vi "draw_time_stamp.vi"(8 "error in (no error)":errorcluster, 11 "Image in":refnum<class "Image.lvclass">) -> (0 "error out":errorcluster, 3 "Image out":refnum<class "Image.lvclass">)   [LabVIEW 2010, in "Image.lvclass"]
uses:
  Image.lvclass
  <vilib>/vision/Image Controls.llb/IMAQ Image.ctl
  ErrorController/ErrorController/class_data.vi
  ErrorController/ErrorController/ErrorController.lvclass
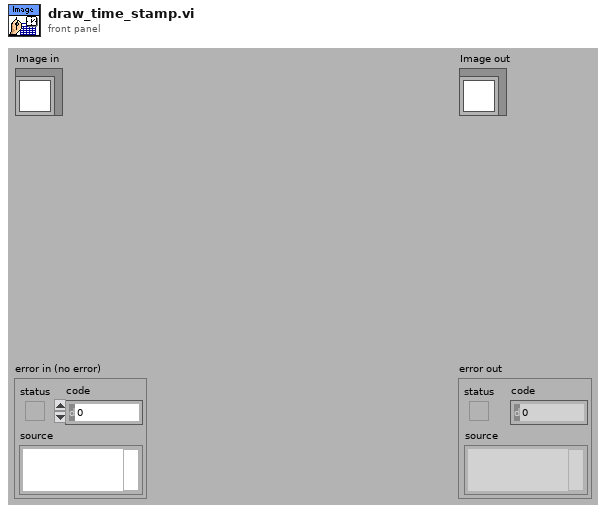
[diagram p1: front panel]
types:
  T1 = cluster{"Desired Font (Application)":enum16{"User-specified Font", "Application Font", "System Font", "Dialog Font"}, "[User-specified Font]":cluster{"Font Name":string, "Size":i16, "Strikeout?":bool, "Italic?":bool, "Underline?":bool, "Outline?":bool, "Shadow?":bool, "Bold?":bool, "Rotation Angle":dbl}, "Horizontal Alignment":i16, "Vertical Alignment":i16}
  T2 = typedef "IMAQ Image.ctl" = refnum<image>
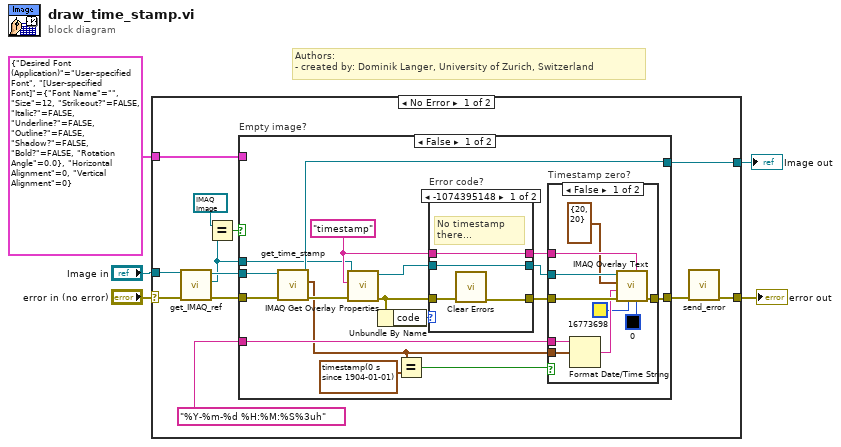
[diagram p0: block diagram]
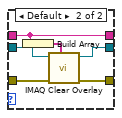
[diagram p3: hidden frame]
diagram:
  # "Authors: \n- created by: Dominik Langer, University of Zurich, Switzerland"
  n1 = case shown="No Error" "error in (no error)" {
    selector: "error in (no error)" -> [w16 w59]
    tunnel: [w7 w59] -> w4
    tunnel: [w17 w58] -> w2
    tunnel: "Image in" -> [w14 w58]
    tunnel: T1 {"Desired Font (Application)"=enum."User-specified Font", "[User-specified Font]"={"Font Name"="", "Size"=12, "Strikeout?"=FALSE, "Italic?"=FALSE, "Underline?"=FALSE, "Outline?"=FALSE, "Shadow?"=FALSE, "Bold?"=FALSE, "Rotation Angle"=0.0}, "Horizontal Alignment"=0, "Vertical Alignment"=0} ("Font, Size & Style") -> [w9 _]
    frame No Error {
      n2 = call-dynamic "get_IMAQ_ref.vi"("error in (no error)"=w16, "Image.lvclass in"=w14) -> ("error out"=w15:errorcluster, "Image"=w11:T2, "Image.lvclass out"=w13:refnum<class "Image.lvclass">)  [unwired: 7 out]
      n3 = Equal?(x=T2 refnum ("y"), y=w11) -> (x = y?=w12:bool)
      n4 = case "Empty image?" shown="False" w12 {
        tunnel: [w23 w56] -> w6
        tunnel: [w34 w57] -> w17
        tunnel: w15 -> [w33 w56]
        tunnel: w13 -> [w32 w57]
        tunnel: w11 -> [w27 _]
        tunnel: w9 -> [_ _]
        tunnel: "%Y-%m-%d %H:%M:%S%3uh" -> [w21 _]
        frame False {
          w30 = "timestamp" ("String")
          n5 = call-dynamic "get_time_stamp.vi"("error in (no error)"=w33, "Image.lvclass in"=w32) -> ("error out"=w26:errorcluster, "timestamp"=w19:timestamp, "Image.lvclass out"=w34:refnum<class "Image.lvclass">)  [unwired: 7 in]
          n6 = call "IMAQ Get Overlay Properties"("error in (no error)"=w26, "Group"=w30, "Image"=w27) -> ("error out"=w29:errorcluster, "Image Out"=w31:T2)  [unwired: 5 out]
          n7 = Unbundle By Name(w29) -> ("code"=w28:i32)
          n8 = Equal?(x=w19, y=timestamp(0 s since 1904-01-01) ("timestamp")) -> (x = y?=w18:bool)
          n9 = case "Error code?" shown="-1074395148" w28 {
            tunnel: [w47 w55] -> w25
            tunnel: [w46 w54] -> w24
            tunnel: w31 -> [w46 w53]
            tunnel: w30 -> [w49 w50]
            tunnel: w29 -> [w48 w51]
            tunnel: [w49 w50] -> w22
            frame -1074395148 {
              # "No timestamp there..."
              n10 = call <vilib>:"Clear Errors.vi"("error in (no error)"=w48) -> ("error out"=w47:errorcluster)  [unwired: 6 out]
            }
            frame Default {
              n11 = Build Array(w50) -> (w52:string[])
              n12 = call "IMAQ Clear Overlay"("Groups"=w52, "error in (no error)"=w51, "Image"=w53) -> ("error out"=w55:errorcluster, "Image Out"=w54:T2)  [unwired: 7 out]
            }
          }
          n13 = case "Timestamp zero?" shown="False" w18 {
            tunnel: w25 -> [w44 w45]
            tunnel: w24 -> [w43 _]
            tunnel: [w42 w45] -> w23
            tunnel: w22 -> [w41 _]
            tunnel: w19 -> [w40 _]
            tunnel: w21 -> [w35 _]
            frame False {
              n14 = Format Date/Time String(time format string (%c)=w35, seconds (now)=w40) -> (date/time string=w39:string)  [unwired: 1 in]
              n15 = call "IMAQ Overlay Text"("BG Color (Transparent)"=u32 0 ("Text Color (black)"), "Group"=w41, "Text Color (black)"=u32 16773698, "error in (no error)"=w44, "String"=w39, "Origin"=cluster{"X":i32, "Y":i32} {"X"=20, "Y"=20}, "Image"=w43) -> ("error out"=w42:errorcluster)  [unwired: 1 in, 3 out]
            }
            frame True {
              # "Don't draw it..."
            }
          }
        }
        frame True {
        }
      }
      n16 = call "send_error.vi"("error in (no error)"=w6) -> ("error out"=w7:errorcluster)  [unwired: 10 in]
    }
    frame Error {
    }
  }
  "error out" <- w4
  "Image out" <- w2
